vi "BarrettPre.vi"(1 "a":cluster{"Boolean":bool, "Array":u64[]}) -> (0 "mu":cluster{"Boolean":bool, "Array":u64[]})   [LabVIEW 2023]
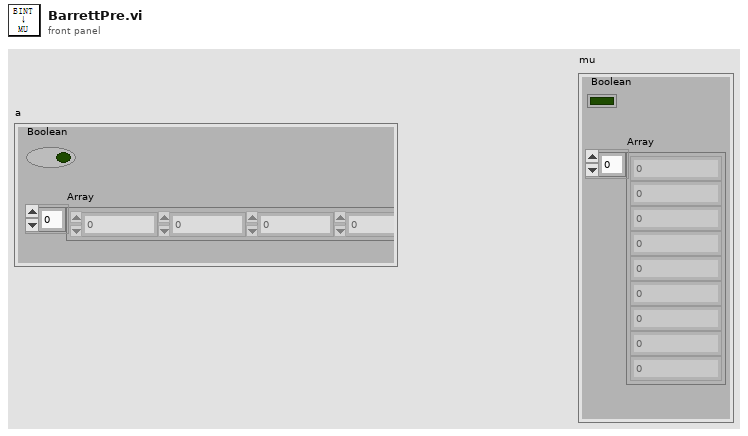
[diagram p1: front panel]
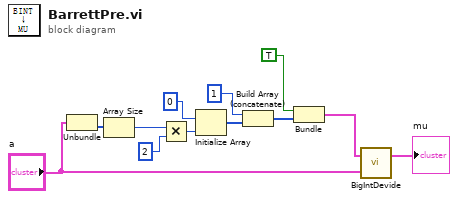
[diagram p0: block diagram]
diagram:
  n1 = Unbundle("a") -> ("Array"=w12:u64[])  [unwired: 1 out]
  n2 = Array Size(array=w12) -> (size(s)=w11:i32)
  n3 = Multiply(x=w11, y=2) -> (x*y=w2:i32)
  n4 = Initialize Array(u64 0, w2) -> (w8:u64[])
  n5 = Build Array (concatenate)(u64 1, w8) -> (w7:u64[])
  n6 = Bundle(TRUE, w7) -> (w5:cluster{bool, u64[]})  [unwired: 1 in]
  n7 = call "BigIntDevide.vi"("b"="a", "a"=w5) -> ("a / b"=→"mu":cluster{"Boolean":bool, "Array":u64[]})  [unwired: 1 out]
